vi "Write Wrap.vi"(8 "error in (no error)":errorcluster, 10 "Wrap":bool, 11 "Cursor in":refnum<class "Cursor.lvclass">) -> (0 "error out":errorcluster, 3 "Cursor out":refnum<class "Cursor.lvclass">)   [LabVIEW 2019, in "RT_Game.lvlib" / "Cursor.lvclass"]
uses:
  Cursor.lvclass
  Cursor.lvclass/Cursor.ctl
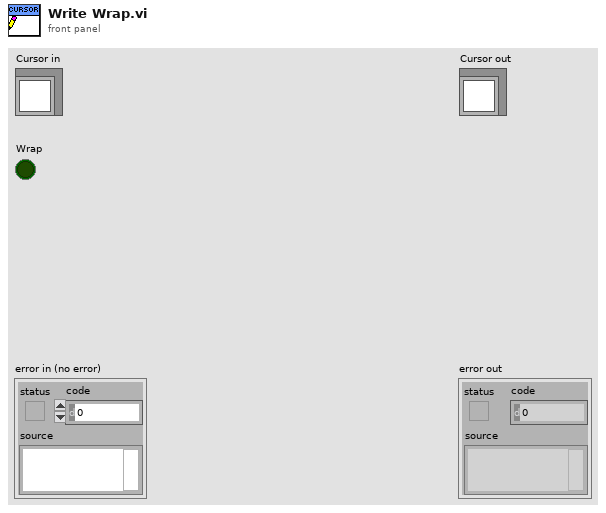
[diagram p1: front panel]
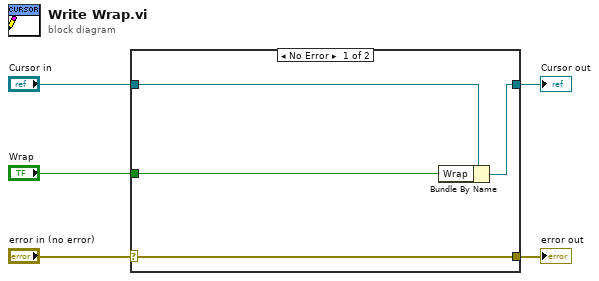
[diagram p0: block diagram]
diagram:
  n1 = case shown="No Error" "error in (no error)" {
    selector: "error in (no error)" -> [w9 w10]
    tunnel: [w9 w10] -> w4
    tunnel: [w7 w11] -> w2
    tunnel: "Cursor in" -> [w8 w11]
    tunnel: "Wrap" -> [w6 _]
    frame No Error {
      n2 = Bundle By Name(cluster=w8, "Wrap"=w6) -> (w7:refnum<class "Cursor.lvclass">)
    }
    frame Error {
    }
  }
  "error out" <- w4
  "Cursor out" <- w2
